vi "scaler_digitial_64channels_example.vi"(8 "PresetValues_Scaler":u32[](array[numeric])=[0, 0, 0, 0, 0, 0, 0, 0, 0, 0, 0, 0, 0, 0, 0, 0, 0, 0, 0, 0, 0, 0, 0, 0, 0, 0, 0, 0, 0, 0, 0, 0, 0, 0, 0, 0, 0, 0, 0, 0, 0, 0, 0, 0, 0, 0, 0, 0, 0, 0, 0, 0, 0, 0, 0, 0, 0, 0, 0, 0, 0, 0, 0, 0], 9 "OneShot_Scaler":bool, 10 "Gate_Scaler":bool[](array[boolean])=[FALSE, FALSE, FALSE, FALSE, FALSE, FALSE, FALSE, FALSE, FALSE, FALSE, FALSE, FALSE, FALSE, FALSE, FALSE, FALSE, FALSE, FALSE, FALSE, FALSE, FALSE, FALSE, FALSE, FALSE, FALSE, FALSE, FALSE, FALSE, FALSE, FALSE, FALSE, FALSE, FALSE, FALSE, FALSE, FALSE, FALSE, FALSE, FALSE, FALSE, FALSE, FALSE, FALSE, FALSE, FALSE, FALSE, FALSE, FALSE, FALSE, FALSE, FALSE, FALSE, FALSE, FALSE, FALSE, FALSE, FALSE, FALSE, FALSE, FALSE, FALSE, FALSE, FALSE, FALSE], 11 "Enable_Scaler":bool) -> (0 "Counter_Scaler":u32[](array[numeric]), 3 "Done_Scaler":bool)   [LabVIEW 2020]
uses:
  <vilib>/Platform/TimedLoop/XDataNode/timing_clust.ctl
  <vilib>/Platform/TimedLoop/XDataNode/nitl_modes.ctl
  <vilib>/Platform/TimedLoop/XDataNode/wakeup.ctl
  <vilib>/rvi/Emulation/niFpgaGetClockAttributes.vi
  <vilib>/rvi/Emulation/niFpgaSctlEmulationGetInTimedLoop.vi
  <vilib>/rvi/Emulation/niFpgaEmulationReportErrorSimple.vi
  <vilib>/rvi/eio/common/nirviEmuTemplateMethod_errors.vi
  <vilib>/rvi/Emulation/niFpgaProcessEmulError.vi
  <vilib>/rvi/Emulation/niFpgaCriticalErrorInLSC.vi
  <vilib>/eio/EIONode/EIONode.xnode
  <vilib>/Platform/TimedLoop/XDataNode/XDataNode.xnode
  <vilib>/Platform/TimedLoop/XDataNode/XDNodeRunTimeDep.lvlib
  lib/Scaler-EPICS/scaler.lvlib
panel:
  out "Pulse_Scaler":u64
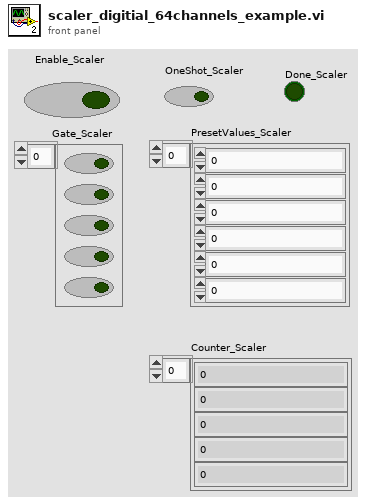
[diagram p1: front panel]
types:
  T1 = typedef "XDNodeRunTimeDep.lvlib/timing_clust.ctl" = cluster{"Expected End [f-1]":u64, "Actual End [f-1]":u64, "Finished Late? [f-1]":bool, "Expected End [i-1]":u64, "Actual End [i-1]":u64, "Finished Late? [i-1]":bool, "Expected Start [i]":u64, "Actual Start [i]":u64, "Expected Start [f]":u64, "Actual Start [f]":u64, "Source Name":string, "Structure Name":string, "Period":i64, "Deadline":i64, "Offset":i64, "Start":i64, "Priority":i32, "Timeout":i32, "Mode":T2, "Wakeup Reason":T3, "Error":errorcluster, "Source Type":string, "Secondary Source Type":string, "Global End Time":u64, "Global Start Time":u64, "Frame Duration":u64, "Iteration Duration":u64, "Assigned CPU":i32, "I/O Scan Engine Mode":u32}
  T2 = typedef "XDNodeRunTimeDep.lvlib/nitl_modes.ctl" = enum32{"No Change", "Process missed periods, maintain original phase", "Discard missed periods, maintain original phase", "Process missed periods, ignore original phase", "Discard missed periods, ignore original phase"}
  T3 = typedef "XDNodeRunTimeDep.lvlib/wakeup.ctl" = enum32{"Normal", "Aborted", "Asynchronous wakeup", "Timing source error", "Timed loop error", "Timeout"}
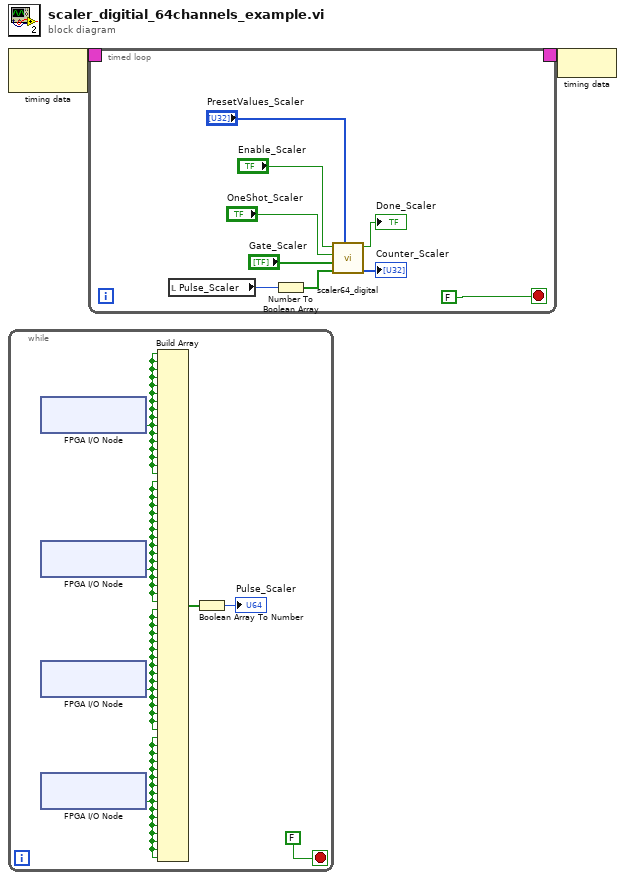
[diagram p0: block diagram]
diagram:
  n1 = node-c288() -> (w2:T1)  [unwired: 1 in]
  n2 = while {
    stop <- FALSE stop-if-true
    n3 = xnode "FPGA I/O Node"() -> ("Mod2/DIO0"=w6:bool)  [unwired: 1 in, 1 out]
    n4 = xnode "FPGA I/O Node"() -> ("Mod2/DIO1"=w5:bool)  [unwired: 1 in, 1 out]
    n5 = xnode "FPGA I/O Node"() -> ("Mod2/DIO2"=w4:bool)  [unwired: 1 in, 1 out]
    n6 = xnode "FPGA I/O Node"() -> ("Mod2/DIO3"=w3:bool)  [unwired: 1 in, 1 out]
    n7 = Build Array(w6, w6, w6, w6, w6, w6, w6, w6, w6, w6, w6, w6, w6, w6, w6, w6, w5, w5, w5, w5, w5, w5, w5, w5, w5, w5, w5, w5, w5, w5, w5, w5, w4, w4, w4, w4, w4, w4, w4, w4, w4, w4, w4, w4, w4, w4, w4, w4, w3, w3, w3, w3, w3, w3, w3, w3, w3, w3, w3, w3, w3, w3, w3, w3) -> (w8:bool[])
    n8 = Boolean Array To Number(Boolean array=w8) -> (number=→"Pulse_Scaler":u64)
  }
  n9 = timed-loop {
    timing: w2 -> [_]
    timing-out: [_] -> w1
    stop <- FALSE stop-if-true
    n10 = local read "Pulse_Scaler"() -> (w17:u64)
    n11 = Number To Boolean Array(number=w17) -> (Boolean array=w12:bool[])
    n12 = call "scaler64_digital.vi"("PresetValues_SCALER"="PresetValues_Scaler", "Pulse_SCALER"=w12, "Gate_SCALER"="Gate_Scaler", "OneShot_SCALER"="OneShot_Scaler", "Enable_SCALER"="Enable_Scaler") -> ("Counter_SCALER"=→"Counter_Scaler":u32[], "Done_SCALER"=→"Done_Scaler":bool)  [unwired: 5 in]
  }
  n13 = node-c288(w1) -> ()
